vi "Angle_test.vi"() -> ()   [LabVIEW 2020]
uses:
  <vilib>/Platform/TimedLoop/XDataNode/timing_clust.ctl
  <vilib>/Platform/TimedLoop/XDataNode/nitl_modes.ctl
  <vilib>/Platform/TimedLoop/XDataNode/wakeup.ctl
  <vilib>/Platform/TimedLoop/XDataNode/XDataNode.xnode
  <vilib>/Platform/TimedLoop/XDataNode/XDNodeRunTimeDep.lvlib
panel:
  out "Encode_Swing":dbl
  out "Encode_Boom":dbl
  in  "Open_Loop U":T1
  out "Encode_Stick":dbl
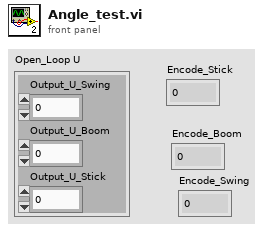
[diagram p1: front panel]
types:
  T1 = cluster{"Output_U_Swing":dbl, "Output_U_Boom":dbl, "Output_U_Stick":dbl}
  T2 = typedef "XDNodeRunTimeDep.lvlib/timing_clust.ctl" = cluster{"Expected End [f-1]":u64, "Actual End [f-1]":u64, "Finished Late? [f-1]":bool, "Expected End [i-1]":u64, "Actual End [i-1]":u64, "Finished Late? [i-1]":bool, "Expected Start [i]":u64, "Actual Start [i]":u64, "Expected Start [f]":u64, "Actual Start [f]":u64, "Source Name":string, "Structure Name":string, "Period":i64, "Deadline":i64, "Offset":i64, "Start":i64, "Priority":i32, "Timeout":i32, "Mode":T3, "Wakeup Reason":T4, "Error":errorcluster, "Source Type":string, "Secondary Source Type":string, "Global End Time":u64, "Global Start Time":u64, "Frame Duration":u64, "Iteration Duration":u64, "Assigned CPU":i32, "I/O Scan Engine Mode":u32}
  T3 = typedef "XDNodeRunTimeDep.lvlib/nitl_modes.ctl" = enum32{"No Change", "Process missed periods, maintain original phase", "Discard missed periods, maintain original phase", "Process missed periods, ignore original phase", "Discard missed periods, ignore original phase"}
  T4 = typedef "XDNodeRunTimeDep.lvlib/wakeup.ctl" = enum32{"Normal", "Aborted", "Asynchronous wakeup", "Timing source error", "Timed loop error", "Timeout"}
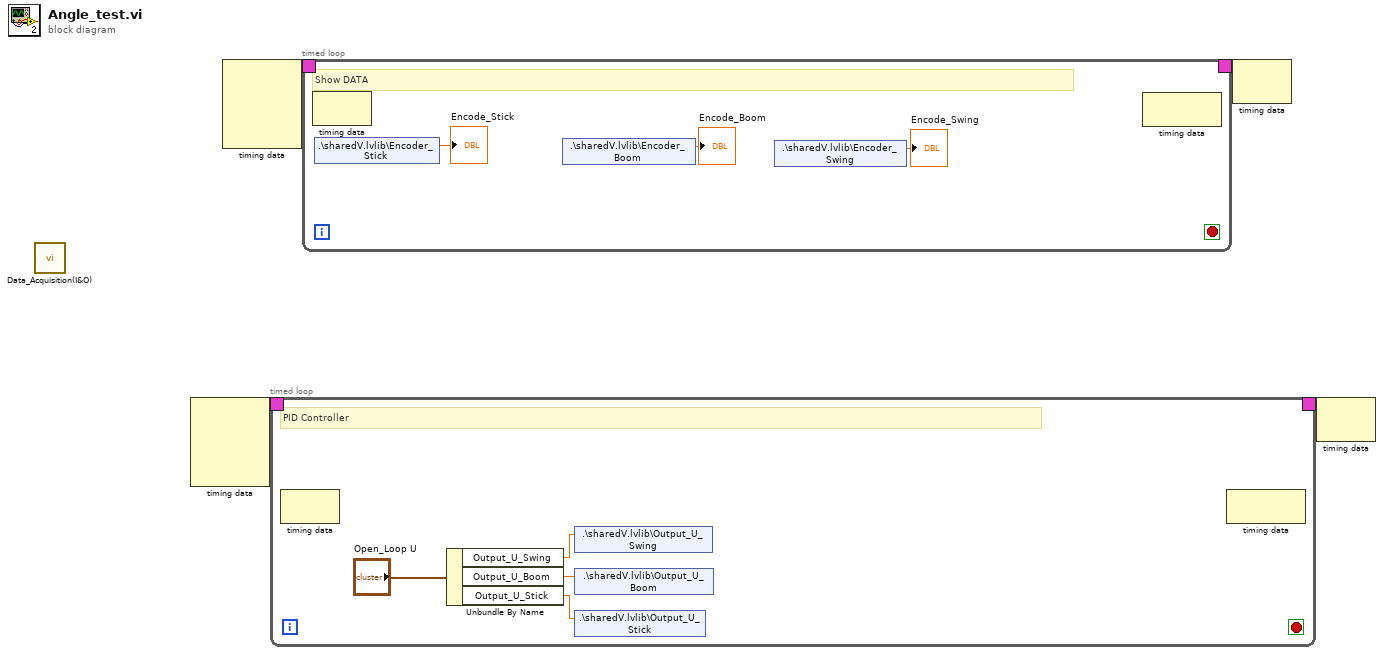
[diagram p0: block diagram]
diagram:
  n1 = call "Data_Acquisition(I&O).vi"() -> ()  [unwired: 12 in]
  n2 = node-c288() -> (w2:T2)  [unwired: 4 in]
  n3 = node-c288() -> (w4:T2)  [unwired: 4 in]
  n4 = timed-loop {
    timing: w2 -> [_]
    timing-out: [_] -> w1
    stop <- _ stop-if-true
    # "PID Controller"
    n5 = node-c288() -> ()  [unwired: 1 in, 1 out]
    n6 = Unbundle By Name("Open_Loop U") -> ("Output_U_Swing"=w8:dbl, "Output_U_Boom"=w7:dbl, "Output_U_Stick"=w6:dbl)
    n7 = shared-variable ".\\sharedV.lvlib\\Output_U_Swing"(w8) -> ()  [unwired: 1 in, 1 out]
    n8 = shared-variable ".\\sharedV.lvlib\\Output_U_Boom"(w7) -> ()  [unwired: 1 in, 1 out]
    n9 = shared-variable ".\\sharedV.lvlib\\Output_U_Stick"(w6) -> ()  [unwired: 1 in, 1 out]
    n10 = node-c288() -> ()  [unwired: 1 in, 1 out]
  }
  n11 = timed-loop {
    timing: w4 -> [_]
    timing-out: [_] -> w3
    stop <- _ stop-if-true
    # "Show DATA"
    n12 = node-c288() -> ()  [unwired: 1 in, 1 out]
    n13 = shared-variable ".\\sharedV.lvlib\\Encoder_Stick"() -> (→"Encode_Stick":dbl)  [unwired: 1 in, 1 out]
    n14 = shared-variable ".\\sharedV.lvlib\\Encoder_Boom"() -> (→"Encode_Boom":dbl)  [unwired: 1 in, 1 out]
    n15 = shared-variable ".\\sharedV.lvlib\\Encoder_Swing"() -> (→"Encode_Swing":dbl)  [unwired: 1 in, 1 out]
    n16 = node-c288() -> ()  [unwired: 1 in, 1 out]
  }
  n17 = node-c288(w3) -> ()  [unwired: 1 out]
  n18 = node-c288(w1) -> ()  [unwired: 1 out]
